vi "GetUserFramePosition.vi"(8 "group":i32, 9 "userFrame":i32, 10 "Snpx":refnum<k24>, 11 "error in":errorcluster) -> (0 "UserTool":i16, 1 "Cartesian position":T1, 2 "JointsPosition":dbl[](array[numeric]), 3 "error out":errorcluster)   [LabVIEW 2013, in "UnderAutomation.Fanuc.lvlib"]
uses:
  UnderAutomation.Fanuc.lvlib
  C:/Users/fg/Documents/Fanuc.vi/LabVIEW_2024/UnderAutomation.Fanuc/lib/UnderAutomation.Fanuc.dll
  LabVIEW_2024/UnderAutomation.Fanuc/lib/UnderAutomation.Fanuc.dll
panel:
  out "UserFrame":i16
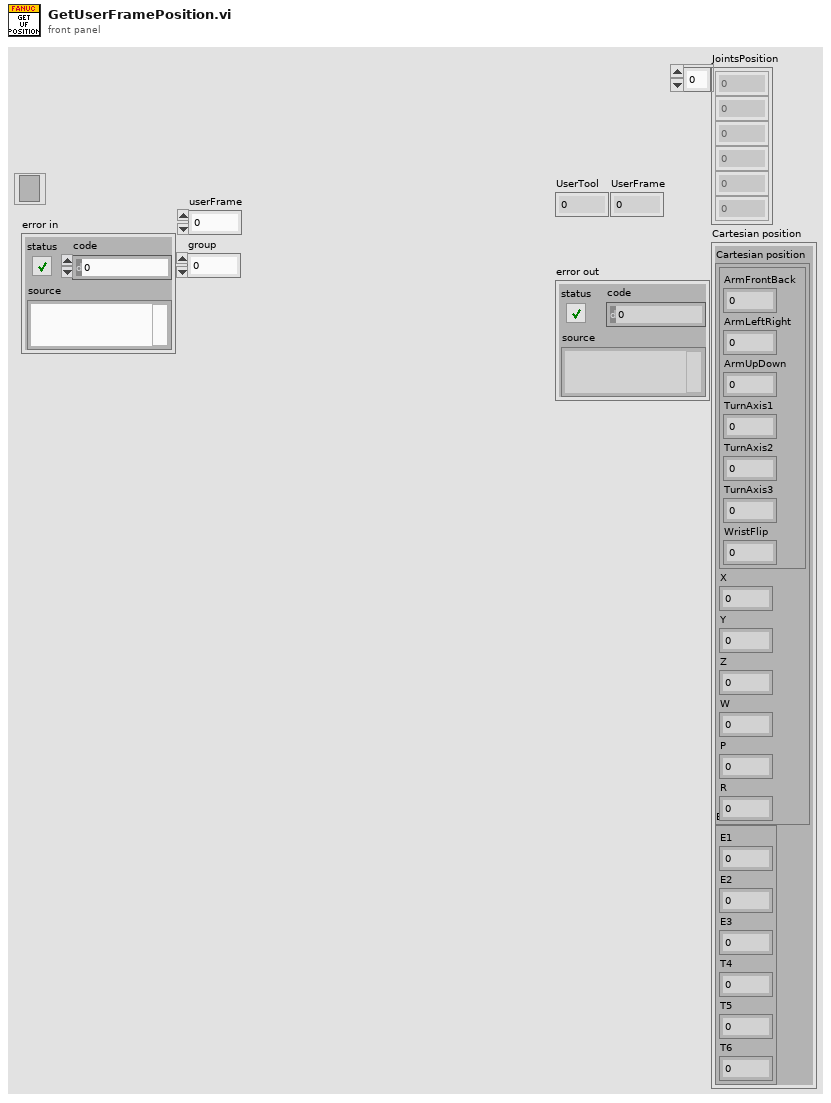
[diagram p1: front panel]
types:
  T1 = cluster{"Cartesian position":cluster{cluster{"ArmFrontBack":i32, "ArmLeftRight":i32, "ArmUpDown":i32, "TurnAxis1":i32, "TurnAxis2":i32, "TurnAxis3":i32, "WristFlip":i32}, "X":dbl, "Y":dbl, "Z":dbl, "W":dbl, "P":dbl, "R":dbl}, "Extension":cluster{"E1":dbl, "E2":dbl, "E3":dbl, "T4":i16, "T5":i16, "T6":i16}}
  T2 = cluster{"Configuration":cluster{"ArmFrontBack":i32, "ArmLeftRight":i32, "ArmUpDown":i32, "TurnAxis1":i32, "TurnAxis2":i32, "TurnAxis3":i32, "WristFlip":i32}, "X":dbl, "Y":dbl, "Z":dbl, "W":dbl, "P":dbl, "R":dbl}
  T3 = cluster{"E1":dbl, "E2":dbl, "E3":dbl, "E3":dbl, "E3":dbl, "E3":dbl}
  T4 = cluster{"Cartesian position":cluster{"Configuration":cluster{"ArmFrontBack":i32, "ArmLeftRight":i32, "ArmUpDown":i32, "TurnAxis1":i32, "TurnAxis2":i32, "TurnAxis3":i32, "WristFlip":i32}, "X":dbl, "Y":dbl, "Z":dbl, "W":dbl, "P":dbl, "R":dbl}, cluster{"E1":dbl, "E2":dbl, "E3":dbl, "E3":dbl, "E3":dbl, "E3":dbl}}
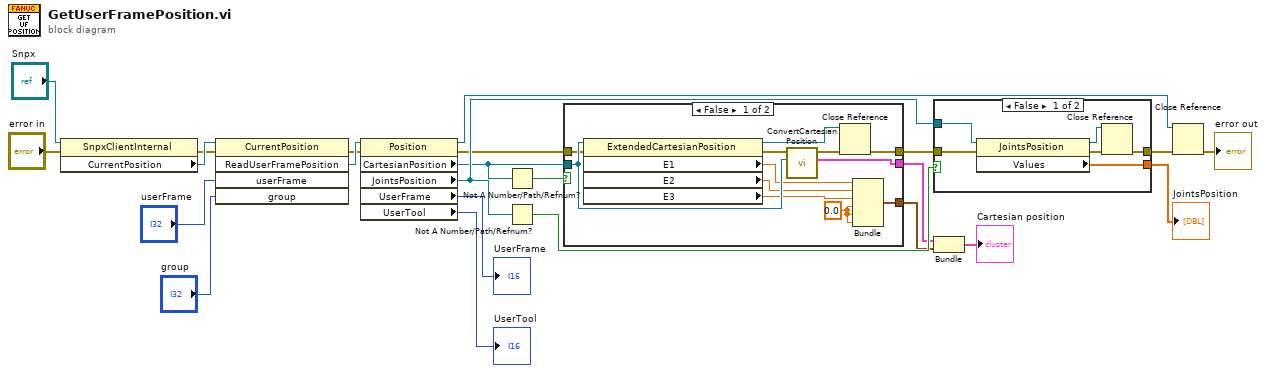
[diagram p0: block diagram]
diagram:
  n1 = property class="SnpxClientInternal"(reference="Snpx", error in="error in") -> (error out=w20:errorcluster, "CurrentPosition"=w21:refnum<k24>)  [unwired: 1 out]
  n2 = invoke class="CurrentPosition" method="ReadUserFramePosition"(reference=w21, error in=w20, "userFrame"="userFrame", "group"="group") -> (error out=w4:errorcluster, "ReadUserFramePosition"=w19:refnum<k24>)  [unwired: 1 in, 3 out]
  n3 = property class="Position"(reference=w19, error in=w4) -> (reference out=w18:refnum<k24>, error out=w7:errorcluster, "CartesianPosition"=w12:refnum<k24>, "JointsPosition"=w14:refnum<k24>, "UserFrame"=→"UserFrame":i16, "UserTool"=→"UserTool":i16)
  n4 = Not A Number/Path/Refnum?(number/path/refnum=w12) -> (NaN/Path/Refnum?=w11:bool)
  n5 = Not A Number/Path/Refnum?(number/path/refnum=w14) -> (NaN/Path/Refnum?=w15:bool)
  n6 = case shown="False" w11 {
    tunnel: w12 -> [w34 _]
    tunnel: [w35 _] -> w10
    tunnel: [w30 _] -> w9
    tunnel: w7 -> [w29 w36]
    tunnel: [w27 w36] -> w6
    frame False {
      w24 = 0.0 ("E3")
      n7 = property class="ExtendedCartesianPosition"(reference=w34, error in=w29) -> (reference out=w28:refnum<k24>, error out=w26:errorcluster, "E1"=w33:dbl, "E2"=w32:dbl, "E3"=w31:dbl)
      n8 = call "ConvertCartesianPosition.vi"("Cartesian position"=w34, "error in (no error)"=w26) -> ("Cartesian position"=w35:T2, "error out"=w25:errorcluster)  [unwired: 8 in]
      n9 = Close Reference(reference=w28, error in (no error)=w25) -> (error out=w27:errorcluster)
      n10 = Bundle("E1"=w33, "E2"=w32, "E3"=w31, "E3"=w24, "E3"=w24, "E3"=w24) -> (w30:T3)  [unwired: 1 in]
    }
    frame True {
    }
  }
  n11 = case shown="False" w15 {
    tunnel: w14 -> [w42 _]
    tunnel: [w41 _] -> w13
    tunnel: w6 -> [w38 w43]
    tunnel: [w37 w43] -> w5
    frame False {
      n12 = property class="JointsPosition"(reference=w42, error in=w38) -> (reference out=w39:refnum<k24>, error out=w40:errorcluster, "Values"=w41:dbl[])
      n13 = Close Reference(reference=w39, error in (no error)=w40) -> (error out=w37:errorcluster)
    }
    frame True {
    }
  }
  "JointsPosition" <- w13
  n14 = Bundle("Cartesian position"=w10, w9) -> (→"Cartesian position":T4)  [unwired: 1 in]
  n15 = Close Reference(reference=w18, error in (no error)=w5) -> (error out=→"error out":errorcluster)
